vi "Max Time Finished.vi"(1 "Max Acceleration":dbl, 2 "Angle Displacement":dbl) -> (0 "Max Time Finished":dbl)   [LabVIEW 2015]
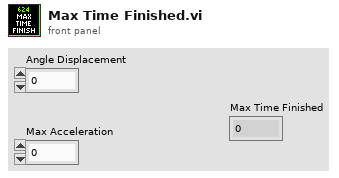
[diagram p1: front panel]
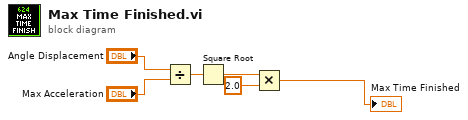
[diagram p0: block diagram]
diagram:
  n1 = Divide(x="Angle Displacement", y="Max Acceleration") -> (x/y=w2:dbl)
  n2 = Square Root(x=w2) -> (sqrt(x)=w6:dbl)
  n3 = Multiply(x=w6, y=2.0) -> (x*y=→"Max Time Finished":dbl)
